vi "BATTERY TEMPERATURE VI.vi"(4 "Numeric Control in":dbl, 6 "Numeric Control 6":dbl, 7 "read buffer":string, 9 "Numeric Control 7":dbl, 10 "Numeric Control 8":dbl, 11 "Numeric Control 9":dbl) -> (0 "Numeric Control out":dbl, 1 "Numeric Control 4":dbl, 2 "Numeric Control 5":dbl, 3 "Numeric Control 10":dbl, 5 "Numeric Control 3":dbl)   [LabVIEW 2016]
panel:
  out "hex integer string 2":string[](array[string])
  out "hex integer string":string[](array[string])
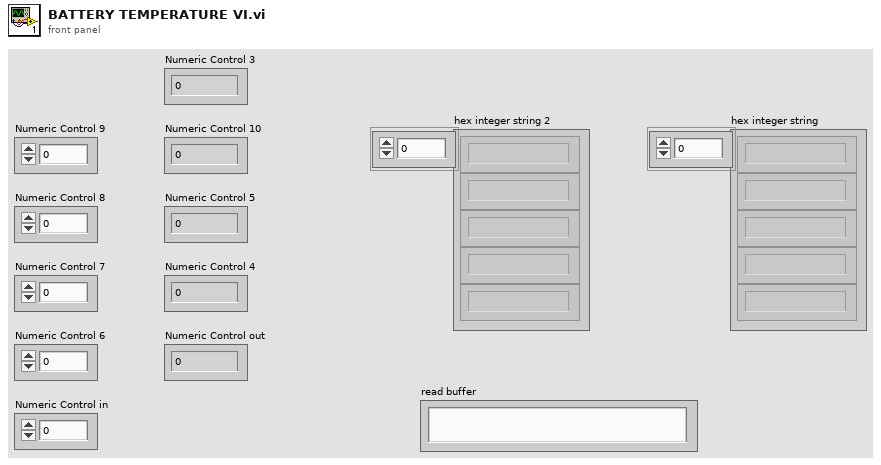
[diagram p1: front panel]
types:
  T1 = cluster{"unsigned byte array[0]":u8, "unsigned byte array[1]":u8, "unsigned byte array[2]":u8, "unsigned byte array[3]":u8, "unsigned byte array[4]":u8, "unsigned byte array[5]":u8, "unsigned byte array[6]":u8, "unsigned byte array[7]":u8, "unsigned byte array[8]":u8}
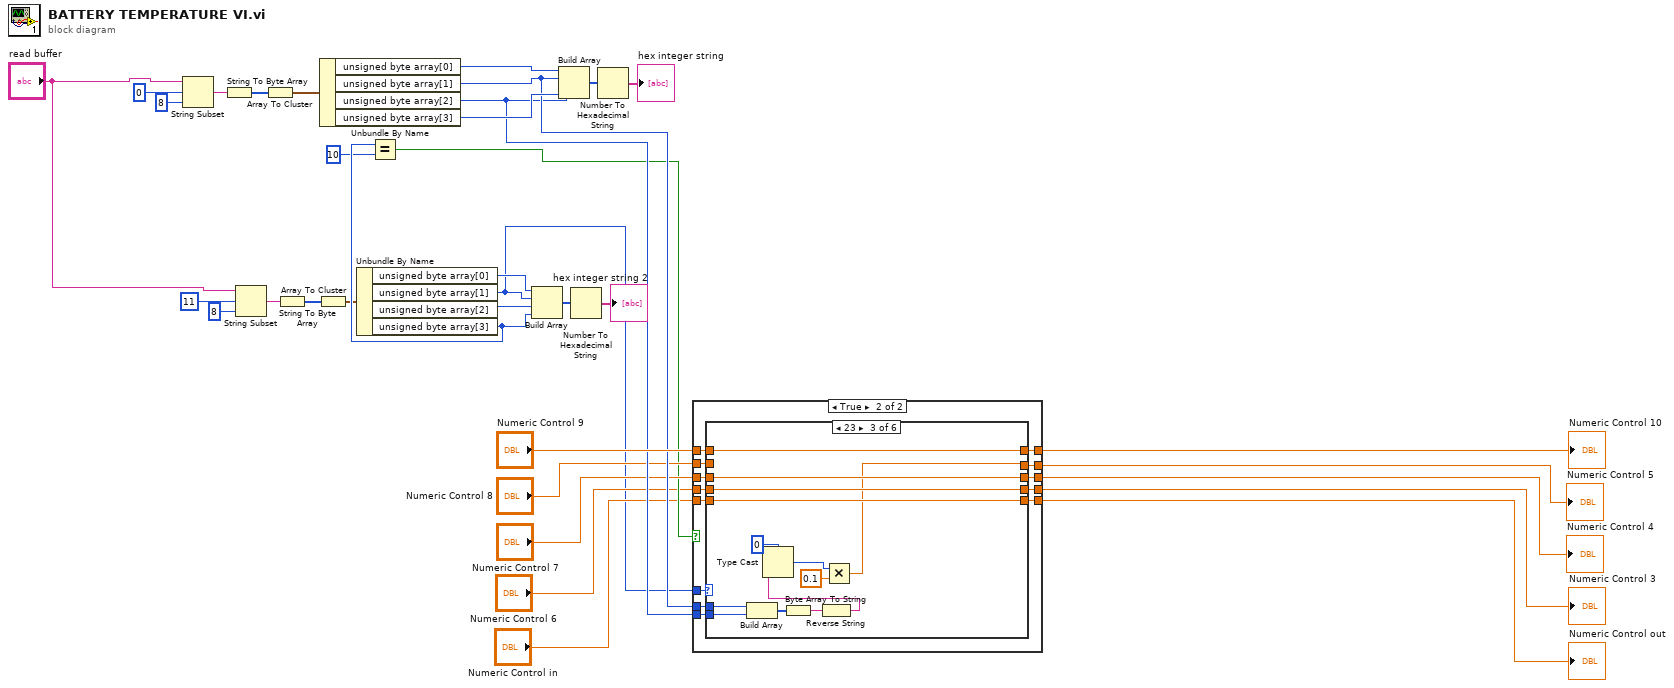
[diagram p0: block diagram]
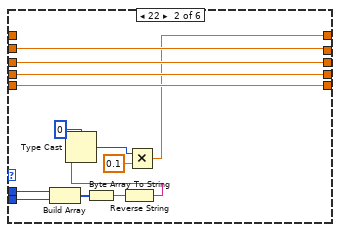
[diagram p4: hidden frame]
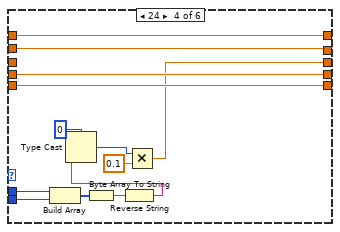
[diagram p5: hidden frame]
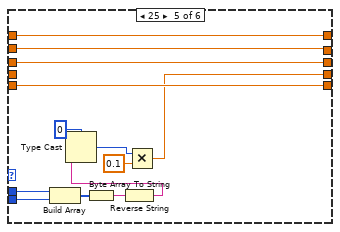
[diagram p6: hidden frame]
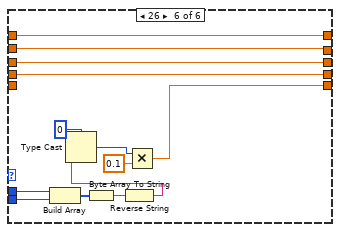
[diagram p7: hidden frame]
diagram:
  n1 = String Subset(string="read buffer", offset (0)=0, length (rest)=8 ("length (rest)")) -> (substring=w20:string)
  n2 = String To Byte Array(string=w20) -> (unsigned byte array=w21:u8[])
  n3 = String Subset(string="read buffer", offset (0)=11, length (rest)=8 ("length (rest)")) -> (substring=w26:string)
  n4 = Array To Cluster(array=w21) -> (cluster=w22:T1)
  n5 = String To Byte Array(string=w26) -> (unsigned byte array=w27:u8[])
  n6 = Array To Cluster(array=w27) -> (cluster=w28:T1)
  n7 = Unbundle By Name(w22) -> ("unsigned byte array[0]"=w32:u8, "unsigned byte array[1]"=w16:u8, "unsigned byte array[2]"=w15:u8, "unsigned byte array[3]"=w33:u8)
  n8 = Unbundle By Name(w28) -> ("unsigned byte array[0]"=w30:u8, "unsigned byte array[1]"=w2:u8, "unsigned byte array[2]"=w31:u8, "unsigned byte array[3]"=w35:u8)
  n9 = Equal?(x=w35, y=u32 10) -> (x = y?=w10:bool)
  n10 = Build Array(w30, w2, w31, w35) -> (w29:u8[])
  n11 = Build Array(w32, w16, w15, w33) -> (w23:u8[])
  n12 = Number To Hexadecimal String(2:w29) -> (0:→"hex integer string 2":string[])  [unwired: 1 in]
  n13 = Number To Hexadecimal String(2:w23) -> (0:→"hex integer string":string[])  [unwired: 1 in]
  n14 = case shown="True" w10 {
    tunnel: "Numeric Control 9" -> [w40 w53]
    tunnel: w16 -> [_ w52]
    tunnel: w15 -> [_ w51]
    tunnel: w2 -> [_ w50]
    tunnel: "Numeric Control 7" -> [w38 w49]
    tunnel: "Numeric Control 8" -> [w39 w48]
    tunnel: [w40 w47] -> w9
    tunnel: [w39 w46] -> w12
    tunnel: [w38 w45] -> w11
    tunnel: "Numeric Control 6" -> [w37 w44]
    tunnel: [w37 w43] -> w7
    tunnel: "Numeric Control in" -> [w36 w42]
    tunnel: [w36 w41] -> w5
    frame False {
    }
    frame True {
      n15 = case shown="23" w50 {
        tunnel: w52 -> [_ w71 w84 w97 w110 w123]
        tunnel: w51 -> [_ w70 w83 w96 w109 w122]
        tunnel: w53 -> [w56 _ w73 w86 w99 w112]
        tunnel: w49 -> [w57 w62 w76 _ w101 w114]
        tunnel: w48 -> [w58 w63 _ w89 w102 w115]
        tunnel: [w56 w59 w73 w86 w99 w112] -> w47
        tunnel: [w58 w63 w72 w89 w102 w115] -> w46
        tunnel: [w57 w62 w76 w85 w101 w114] -> w45
        tunnel: w44 -> [w55 w61 w75 w88 _ w113]
        tunnel: [w55 w61 w75 w88 w98 w113] -> w43
        tunnel: w42 -> [w54 w60 w74 w87 w100 _]
        tunnel: [w54 w60 w74 w87 w100 w111] -> w41
        frame 0, Default {
        }
        frame 22 {
          n16 = Build Array(w71, w70) -> (w69:u8[])
          n17 = Byte Array To String(unsigned byte array=w69) -> (string=w68:string)
          n18 = Reverse String(1:w68) -> (0:w67:string)
          n19 = Type Cast(type=i16 0, x=w67) -> (*(type *) &x=w64:i16)
          n20 = Multiply(x=w64, y=0.1) -> (x*y=w59:dbl)
        }
        frame 23 {
          n21 = Build Array(w84, w83) -> (w82:u8[])
          n22 = Byte Array To String(unsigned byte array=w82) -> (string=w81:string)
          n23 = Reverse String(1:w81) -> (0:w80:string)
          n24 = Type Cast(type=i16 0, x=w80) -> (*(type *) &x=w77:i16)
          n25 = Multiply(x=w77, y=0.1) -> (x*y=w72:dbl)
        }
        frame 24 {
          n26 = Build Array(w97, w96) -> (w95:u8[])
          n27 = Byte Array To String(unsigned byte array=w95) -> (string=w94:string)
          n28 = Reverse String(1:w94) -> (0:w93:string)
          n29 = Type Cast(type=i16 0, x=w93) -> (*(type *) &x=w90:i16)
          n30 = Multiply(x=w90, y=0.1) -> (x*y=w85:dbl)
        }
        frame 25 {
          n31 = Build Array(w110, w109) -> (w108:u8[])
          n32 = Byte Array To String(unsigned byte array=w108) -> (string=w107:string)
          n33 = Reverse String(1:w107) -> (0:w106:string)
          n34 = Type Cast(type=i16 0, x=w106) -> (*(type *) &x=w103:i16)
          n35 = Multiply(x=w103, y=0.1) -> (x*y=w98:dbl)
        }
        frame 26 {
          n36 = Build Array(w123, w122) -> (w121:u8[])
          n37 = Byte Array To String(unsigned byte array=w121) -> (string=w120:string)
          n38 = Reverse String(1:w120) -> (0:w119:string)
          n39 = Type Cast(type=i16 0, x=w119) -> (*(type *) &x=w116:i16)
          n40 = Multiply(x=w116, y=0.1) -> (x*y=w111:dbl)
        }
      }
    }
  }
  "Numeric Control out" <- w5
  "Numeric Control 3" <- w7
  "Numeric Control 4" <- w11
  "Numeric Control 5" <- w12
  "Numeric Control 10" <- w9
